vi "VisionGlobal.vi"() -> ()   [LabVIEW 2023]
uses:
  <vilib>/Rock Robotics/WPI/ThirdParty/JAS_Junk/TrajLib/TypeDef/POSE2D.ctl
  <vilib>/Rock Robotics/WPI/ThirdParty/JAS_Junk/TrajLib/TypeDef/TRANSLATION2D.ctl
  <vilib>/Rock Robotics/WPI/ThirdParty/JAS_Junk/TrajLib/TypeDef/ROTATION2D.ctl
  <vilib>/Rock Robotics/WPI/ThirdParty/JAS_Junk/TrajLib/Trajectory_Library.lvlib
panel:
  out "Vision_BackRight_LastSecCount":i32=-1
  out "Vision_BackRight_Latency_MS":dbl
  out "Vision_BackRight_HasTarg":bool
  out "Vision_BackRight_NewData":bool
  out "Vision_BackRightTime_Sec":dbl
  out "Vision_BackRightAng_Deg":dbl
  out "Vision_BackRightY_Ft":dbl
  out "Vision_BackRightX_Ft":dbl
  out "Vision Conn BR":bool
  out "Vision Count BR":i32=-1
  out "Vision Err BR":bool
  out "Vision_BackBack_LastSecCount":i32=-1
  out "Vision_BackBack_Latency_MS":dbl
  out "Vision_BackBack_HasTarg":bool
  out "Vision_BackBack_NewData":bool
  out "Vision_BackBackTime_Sec":dbl
  out "Vision_BackBackAng_Deg":dbl
  out "Vision_BackBackY_Ft":dbl
  out "Vision_BackBackX_Ft":dbl
  out "Vision Conn BB":bool
  out "Vision Count BB":i32=-1
  out "Vision Err BB":bool
  out "Vision_MaxAllowedAmbiguity":dbl=0.14
  out "Vision_Right_LastSecCount":i32=-1
  out "Vision_Left_LastSecCount":i32=-1
  out "Vision_Right_Latency_MS":dbl
  out "Vision_Left_Latency_MS":dbl
  out "Vision_Right_HasTarg":bool
  out "Vision_Right_NewData":bool
  out "Vision_Left_HasTarg":bool
  out "Vision_Left_NewData":bool
  out "Vision_LeftTime_Sec":dbl
  out "Vision_RightAng_Deg":dbl
  out "Vision_RightY_Ft":dbl
  out "Vision_RightX_Ft":dbl
  out "Vision_RightTime_Sec":dbl
  out "Vision_LeftAng_Deg":dbl
  out "Vision_LeftY_Ft":dbl
  out "Vision_LeftX_Ft":dbl
  out "VisionFPGATime":dbl
  out "Vision Conn L":bool
  out "Vision Count L":i32=-1
  out "Vision Err L":bool
  out "Vision Conn R":bool
  out "Vision Count R":i32=-1
  out "Vision Err R":bool
  out "Odom Error":bool
  in  "Current ABS Pose":T1={"TRANSLATION"={"X"=0.0, "Y"=0.0}, "ROTATION"={"VALUE"=0.0, "COS"=1.0, "SIN"=0.0}} {"ROTATION"."SIN" format="%13.4f"; "ROTATION"."COS" format="%13.4f"; "ROTATION"."VALUE" format="%13.4f"; "TRANSLATION"."Y" format="%14.3f"; "TRANSLATION"."X" format="%14.3f"}
  in  "Initial ABS Pose":T1={"TRANSLATION"={"X"=0.0, "Y"=0.0}, "ROTATION"={"VALUE"=0.0, "COS"=1.0, "SIN"=0.0}} {"ROTATION"."SIN" format="%13.4f"; "ROTATION"."COS" format="%13.4f"; "ROTATION"."VALUE" format="%13.4f"; "TRANSLATION"."Y" format="%14.3f"; "TRANSLATION"."X" format="%14.3f"}
  # "VISION FRONT LEFT"
  # "VISION FRONT RIGHT"
  # "VISION BACK RIGHT"
  # "VISION BACK BACK"
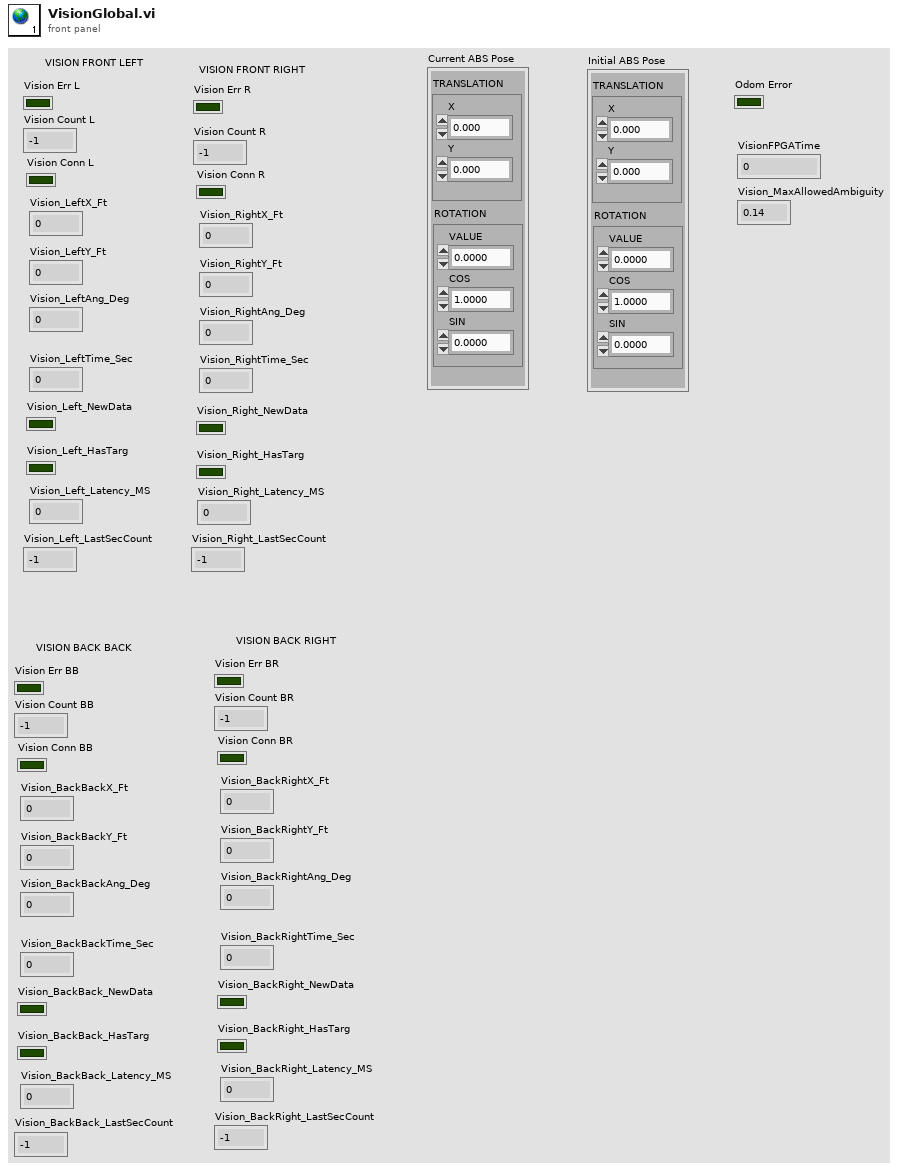
[diagram p1: front panel]
types:
  T1 = typedef "Trajectory_Library.lvlib/POSE2D.ctl" = cluster{"TRANSLATION":T2, "ROTATION":T3}
  T2 = typedef "Trajectory_Library.lvlib/TRANSLATION2D.ctl" = cluster{"X":dbl, "Y":dbl}
  T3 = typedef "Trajectory_Library.lvlib/ROTATION2D.ctl" = cluster{"VALUE":dbl, "COS":dbl, "SIN":dbl}
diagram:
